vi "Add Attributes to Message.vi"(7 "AppInst":refnum<vi>, 8 "error in (no error)":errorcluster, 9 "Original Wiring Rules":T1(array[ring]), 10 "Original Controls":refnum<vi>[](array[refnum])) -> (0 "error out":errorcluster, 1 "Wiring Rules":T1(array[ring]), 2 "Controls":refnum<vi>[](array[refnum]), 3 "Scratch VI Ref":refnum<vi>)   [LabVIEW 2020, in "Message Maker.lvlib"]
uses:
  Message Maker.lvlib
  <vilib>/ErrorRing/Error Ring.xnode
  <vilib>/Utility/miscctls.llb/LVPositionTypeDef.ctl
  <vilib>/Utility/error.llb/Error Cluster From Error Code.vi
panel:
  in  "Cancel":bool
  in  "Next Button":bool
  # "Add attributes to your message class and click Create Message."
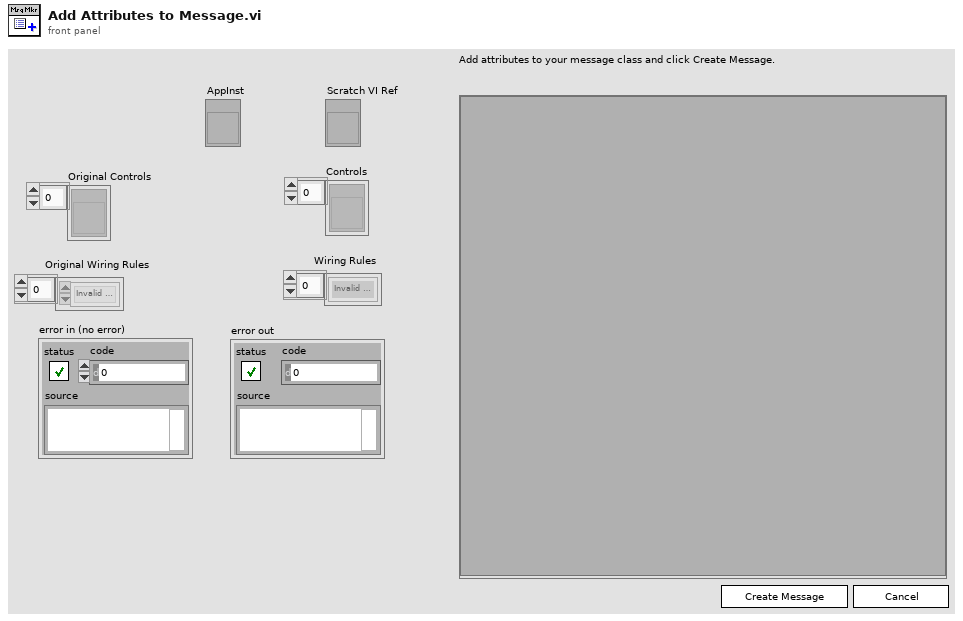
[diagram p1: front panel]
types:
  T1 = enum16{"Invalid Wire Rule", "Required", "Recommended", "Optional", "Dynamic Dispatch"}[]
  T2 = enum16{"Invalid Wire Rule", "Required", "Recommended", "Optional", "Dynamic Dispatch"}
  T3 = typedef "LVPositionTypeDef.ctl" = cluster{"Left":i32, "Top":i32}
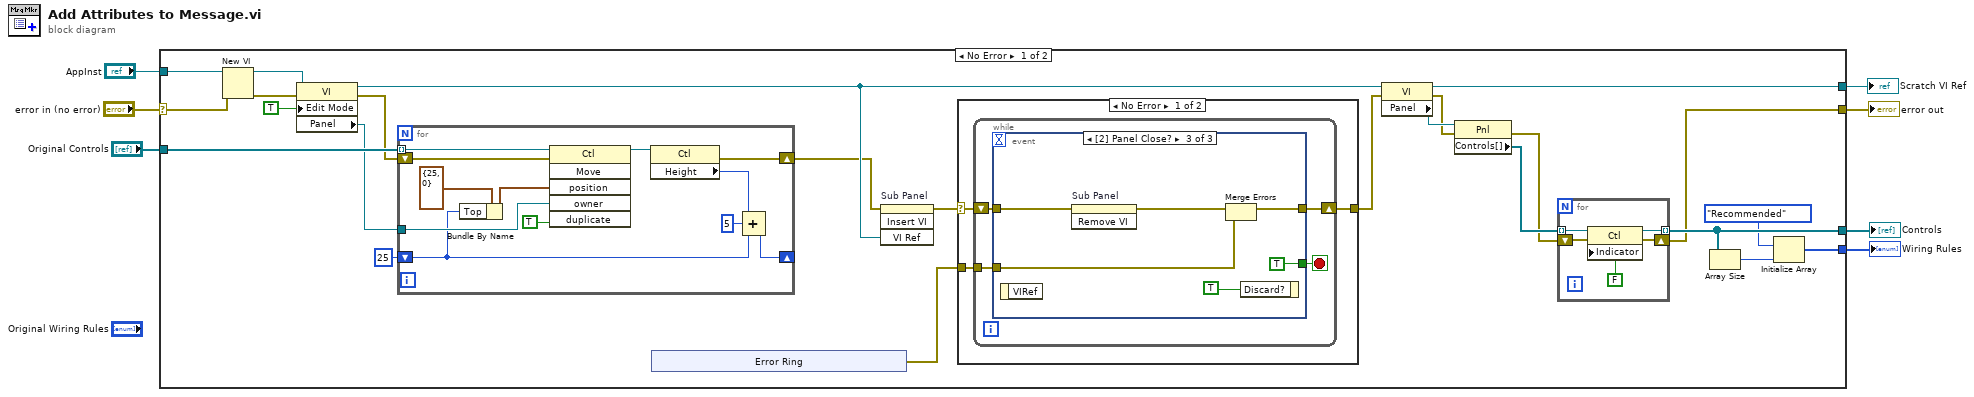
[diagram p0: block diagram]
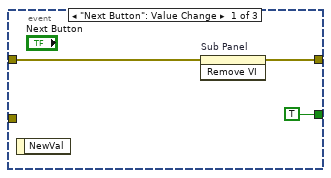
[diagram p2: hidden frame]
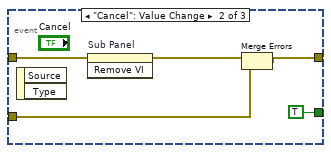
[diagram p3: hidden frame]
diagram:
  n1 = case shown="No Error" "error in (no error)" {
    selector: "error in (no error)" -> [w22 w75]
    tunnel: "AppInst" -> [w25 _]
    tunnel: [w21 w75] -> w5
    tunnel: [w28 _] -> w4
    tunnel: [w24 _] -> w3
    tunnel: [w23 _] -> w2
    tunnel: "Original Controls" -> [w11 _]
    frame No Error {
      n2 = New VI(8:w22, 11:w25) -> (0:w27:errorcluster, 3:w26:refnum<vi>)  [unwired: 5 in]
      n3 = property class="VI"(reference=w26, error in=w27, "Edit Mode"=TRUE ("Edit Mode On Open")) -> (reference out=w29:refnum<vi>, error out=w10:errorcluster, "Panel"=w8:refnum<vi>)
      n4 = for {
        tunnel: w11 -> [w43] mode=indexing
        shift-right: [w33] -> w9
        shift-left: w10 -> [w41]
        tunnel: w8 -> [w39]
        shift-right: [w34] -> _
        shift-left: 25 ("Top") -> [w32]
        n5 = Bundle By Name(cluster=T3 {"Left"=25, "Top"=0} ("position"), "Top"=w32) -> (w37:T3)
        n6 = invoke class="Ctl" method="Move"(reference=w43, error in=w41, "position"=w37, "owner"=w39, "duplicate"=TRUE ("Duplicate? (F)")) -> (reference out=w38:refnum<vi>)  [unwired: 1 in, 5 out]
        n7 = property class="Ctl"(reference=w38) -> (error out=w33:errorcluster, "Height"=w36:u32)  [unwired: 1 in, 1 out]
        n8 = Compound Arithmetic op=ADD(w36, u32 5 ("value"), w32) -> (w34:u32)
      }
      n9 = xnode "Error Ring"() -> ("error out"=w20:errorcluster)
      n10 = invoke on="Sub Panel" class="SubPanel" method="Insert VI"(error in=w9, "VI Ref"=w29) -> (error out=w30:errorcluster)  [unwired: 2 in, 3 out]
      n11 = case shown="No Error" w30 {
        selector: w30 -> [w54 w74]
        tunnel: [w55 w74] -> w19
        tunnel: w20 -> [w53 _]
        frame No Error {
          n12 = while {
            tunnel: w53 -> [w57]
            shift-right: [w59] -> w55
            shift-left: w54 -> [w58]
            stop <- w56 stop-if-true
            n13 = event shown="[2] Panel Close?" {
              selector: _ -> [_ _ _]
              dyn-events: _ -> [_ _ _]
              timeout: _ -> [_ _ _]
              tunnel: w58 -> [w62 w67 w73]
              tunnel: [w61 w64 w70] -> w59
              tunnel: w57 -> [_ w65 w71]
              tunnel: [TRUE TRUE TRUE] -> w56
              event "Next Button": Value Change {
                n14 = event-data() -> ()  [unwired: 1 in, 1 out]
                n15 = invoke on="Sub Panel" class="SubPanel" method="Remove VI"(error in=w62) -> (error out=w61:errorcluster)  [unwired: 2 in, 2 out]
              }
              event "Cancel": Value Change {
                n16 = event-data() -> ()  [unwired: 1 in, 2 out]
                n17 = invoke on="Sub Panel" class="SubPanel" method="Remove VI"(error in=w67) -> (error out=w66:errorcluster)  [unwired: 2 in, 2 out]
                n18 = Merge Errors(w66, w65) -> (w64:errorcluster)
              }
              event Panel Close? {
                n19 = event-data() -> ()  [unwired: 1 in, 1 out]
                n20 = invoke on="Sub Panel" class="SubPanel" method="Remove VI"(error in=w73) -> (error out=w72:errorcluster)  [unwired: 2 in, 2 out]
                n21 = Merge Errors(w72, w71) -> (w70:errorcluster)
                n22 = event-data("Discard?"=TRUE) -> ()  [unwired: 1 in, 1 out]
              }
            }
          }
        }
        frame Error {
        }
      }
      n23 = property class="VI"(reference=w29, error in=w19) -> (reference out=w23:refnum<vi>, error out=w15:errorcluster, "Panel"=w18:refnum<vi>)
      n24 = property class="Pnl"(reference=w18, error in=w15) -> (error out=w13:errorcluster, "Controls[]"=w14:refnum<vi>[])  [unwired: 1 out]
      n25 = for {
        tunnel: w14 -> [w48] mode=indexing
        tunnel: [w47] -> w24 mode=indexing
        shift-right: [w45] -> w21
        shift-left: w13 -> [w46]
        n26 = property class="Ctl"(reference=w48, error in=w46, "Indicator"=FALSE) -> (reference out=w47:refnum<vi>, error out=w45:errorcluster)
      }
      n27 = Array Size(array=w24) -> (size(s)=w17:i32)
      n28 = Initialize Array(T2."Recommended" ("Wire Rule"), w17) -> (w28:T1)
    }
    frame Error {
    }
  }
  "error out" <- w5
  "Wiring Rules" <- w4
  "Controls" <- w3
  "Scratch VI Ref" <- w2
